vi "Receive.vi"(8 "error in (no error)":errorcluster, 10 "Transfer Group in":refnum<class "DSF.Engine.Transfer Group.lvclass">, 11 "Transceiver Thread in":refnum<class "Transceiver Thread.lvclass">) -> (0 "error out":errorcluster, 2 "Transfer Group out":refnum<class "DSF.Engine.Transfer Group.lvclass">, 3 "Transceiver Thread out":refnum<class "Transceiver Thread.lvclass">)   [LabVIEW 2017, in "Data Sharing Framework Engine.lvlib" / "Transceiver Thread.lvclass"]
uses:
  Transceiver Thread.lvclass
  old/dsf core/Source/Engine/Classes/Transfer/DSF.Engine.Transfer Group.lvclass
  Transceiver Thread.lvclass/Transceiver Thread.ctl
  Transceiver/Transceiver.lvclass
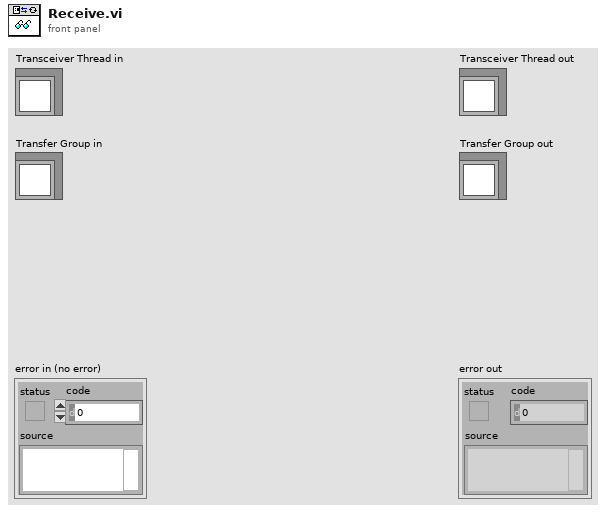
[diagram p1: front panel]
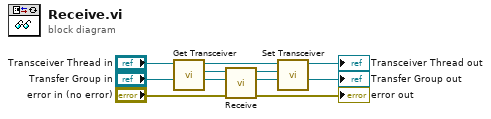
[diagram p0: block diagram]
diagram:
  n1 = call "Get Transceiver.vi"("Transceiver Thread in"="Transceiver Thread in") -> ("Transceiver"=w9:refnum<class "Transceiver.lvclass">, "Transceiver Thread out"=w7:refnum<class "Transceiver Thread.lvclass">)  [unwired: 9 in]
  n2 = call-dynamic "Receive.vi"("error in (no error)"="error in (no error)", "Transfer Group in"="Transfer Group in", "Transceiver in"=w9) -> ("error out"=→"error out":errorcluster, "Transfer Group out"=→"Transfer Group out":refnum<class "DSF.Engine.Transfer Group.lvclass">, "Transceiver out"=w8:refnum<class "Transceiver.lvclass">)  [unwired: 6 in]
  n3 = call "Set Transceiver.vi"("Transceiver"=w8, "Transceiver Thread in"=w7) -> ("Transceiver Thread out"=→"Transceiver Thread out":refnum<class "Transceiver Thread.lvclass">)  [unwired: 9 in]
